vi "USE_THIS_experiment_controller_main_gated.vi"() -> ()   [LabVIEW 2020]
uses:
  <vilib>/Utility/file.llb/Write Delimited Spreadsheet (DBL).vi
  <vilib>/Utility/file.llb/Write To Spreadsheet File (DBL).vi
  <vilib>/Analysis/NI_AALPro.lvlib
  <vilib>/Analysis/2dsp.llb/Integral Method.ctl
  chem-ptch0492/Desktop/IRPD_controler_LV_classic/LeCroy Wave Series/LeCroy Wave Series.lvlib
  <vilib>/Waveform/WDTOps.llb/WDT Get Waveform Subset DBL.vi
panel:
  out "Avg Power / J":dbl format="%#_6f"
  in  "Legacy Mode 2":bool
  in  "Main Tab Control":T1(tab)
  out "Est. total run time / min":dbl
  in  "Legacy Mode":bool
  in  "Scope Trace Tabs":enum32{"Raw Trace", "Avg Traces", "IR Spectrum"}(tab)
  out "Raw Trace":waveform(dbl)(graph)
  out "Avg IR On Chart":waveform(dbl)(graph)
  out "Difference Chart":waveform(dbl)(graph)
  out "Avg IR Off Chart":waveform(dbl)(graph)
  out "Scan Progress":u8(slide) scale=0.0..100.0
  out "IR Spectrum":cluster{dbl[], dbl[]}(graph)
  in  "Laser control":enum32{"Mid IR", "Far IR"}(tab)
  in  "High Position MID / cm-1":dbl
  in  "Step Size MID / cm-1":dbl
  in  "Low Position MID / cm-1":dbl
  in  "Wavenumber MID / cm-1":dbl
  in  "Go to WN MID":bool
  in  "Step Size FAR / cm-1":dbl
  in  "Wavenumber FAR / cm-1":dbl
  in  "High Position FAR / cm-1":dbl
  in  "Low Position FAR / cm-1":dbl
  in  "Go to WN FAR":bool
  in  "Start Scan":bool
  out "Est. time to run / min":dbl
  out "Current Pos / cm-1":dbl
  in  "Number of Sweeps":i32
  in  "Gate Channel (0: Channel 1)":u16(ring) items=["Channel 1", "Channel 2", "Channel 3", "Channel 4", "Memory 1", "Memory 2", "Memory 3", "Memory 4", "Function 1", "Function 2", "Function 3", "Function 4", "Function 5", "Function 6", "Function 7", "Function 8", "Other"]
  in  "Data Channel (0: Channel 1)":u16(ring) items=["Channel 1", "Channel 2", "Channel 3", "Channel 4", "Memory 1", "Memory 2", "Memory 3", "Memory 4", "Function 1", "Function 2", "Function 3", "Function 4", "Function 5", "Function 6", "Function 7", "Function 8", "Other"]
  in  "Laser gate threshold":dbl
  in  "Scope On/Off":bool
  in  "stop":bool
  out "Producer Loop Time / ms":u32
  in  "Auto Setup Scope":bool
  in  "ID Query? (T: Yes)":bool
  in  "Reset? (T: Yes)":bool
  out "Consumer Loop Time / ms":u32
  out "Power / J":dbl
  out "Off queue length":i32
  out "On queue length":i32
  out "Gate Trace":waveform(dbl)(graph)
  out "OPO/OPA motors stationary":bool
  out "OPO/OPA motors reducing errors":bool
  out "OPO/OPA motors scanning red":bool
  out "OPO/OPA motors scanning blue":bool
  # "Ensure that the cursors are gating the peak you are recording the spectrum on if you want a real time spectrum!"
  # "Real Time Controls"
  # "Scanning Controls"
  # "Scan from high to low"
  # "Real Time Controls"
  # "Scanning Controls"
  # "Scan from low to high"
  # "LEAVE THESE ALONE UNLESS YOU KNOW WHAT YOU ARE DOING!"
  # "Gate trace"
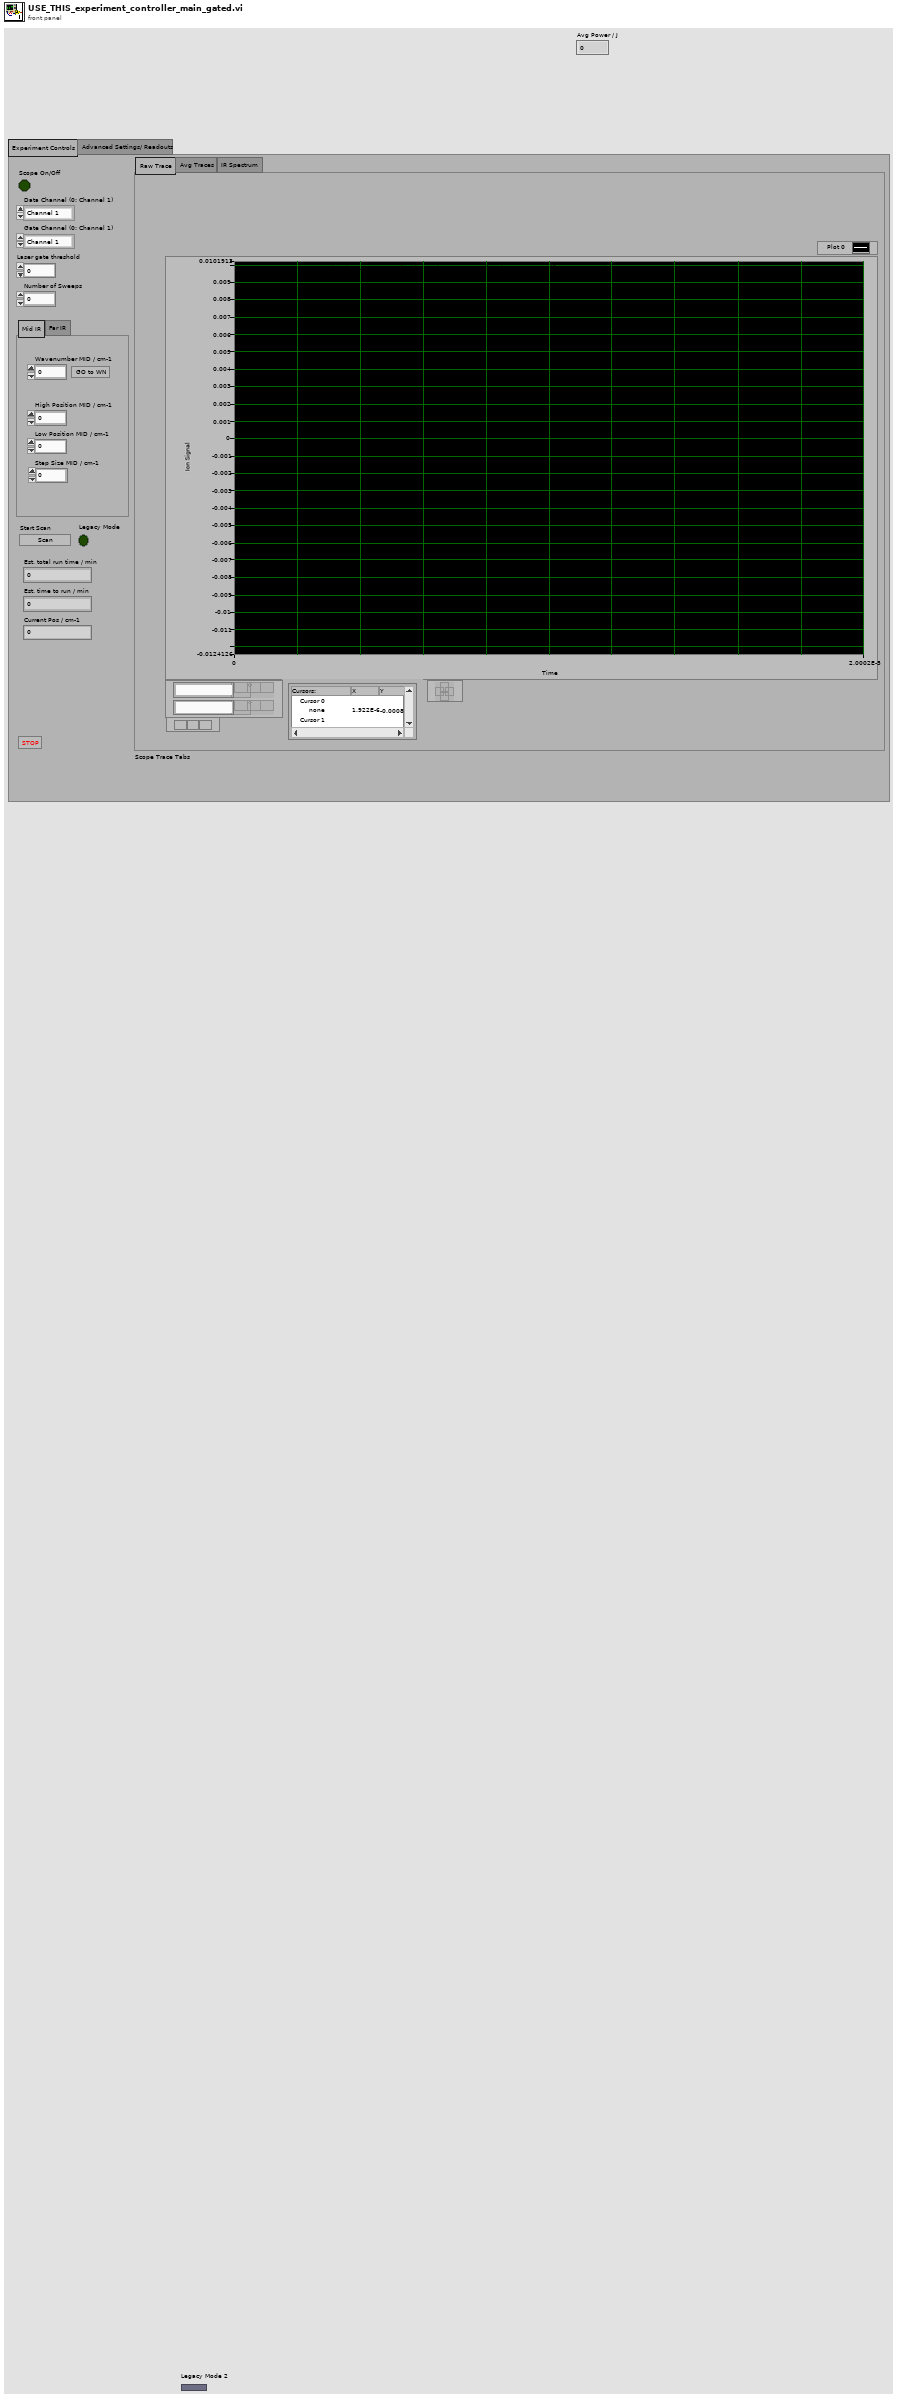
[diagram p1: front panel]
types:
  T1 = enum32{"Experiment Controls", "Advanced Settings/ Readouts"}
  T2 = cluster{"High Position / cm-1":dbl, "Step Size / cm-1":dbl, "Low Position / cm-1":dbl}
  T3 = cluster{"High Position MID / cm-1":dbl, "Step Size MID / cm-1":dbl, "Low Position MID / cm-1":dbl}
  T4 = cluster{"High Position FAR / cm-1":dbl, "Step Size FAR / cm-1":dbl, "Low Position FAR / cm-1 ":dbl}
  T5 = typedef "NI_AALPro.lvlib/Integral Method.ctl" = i32
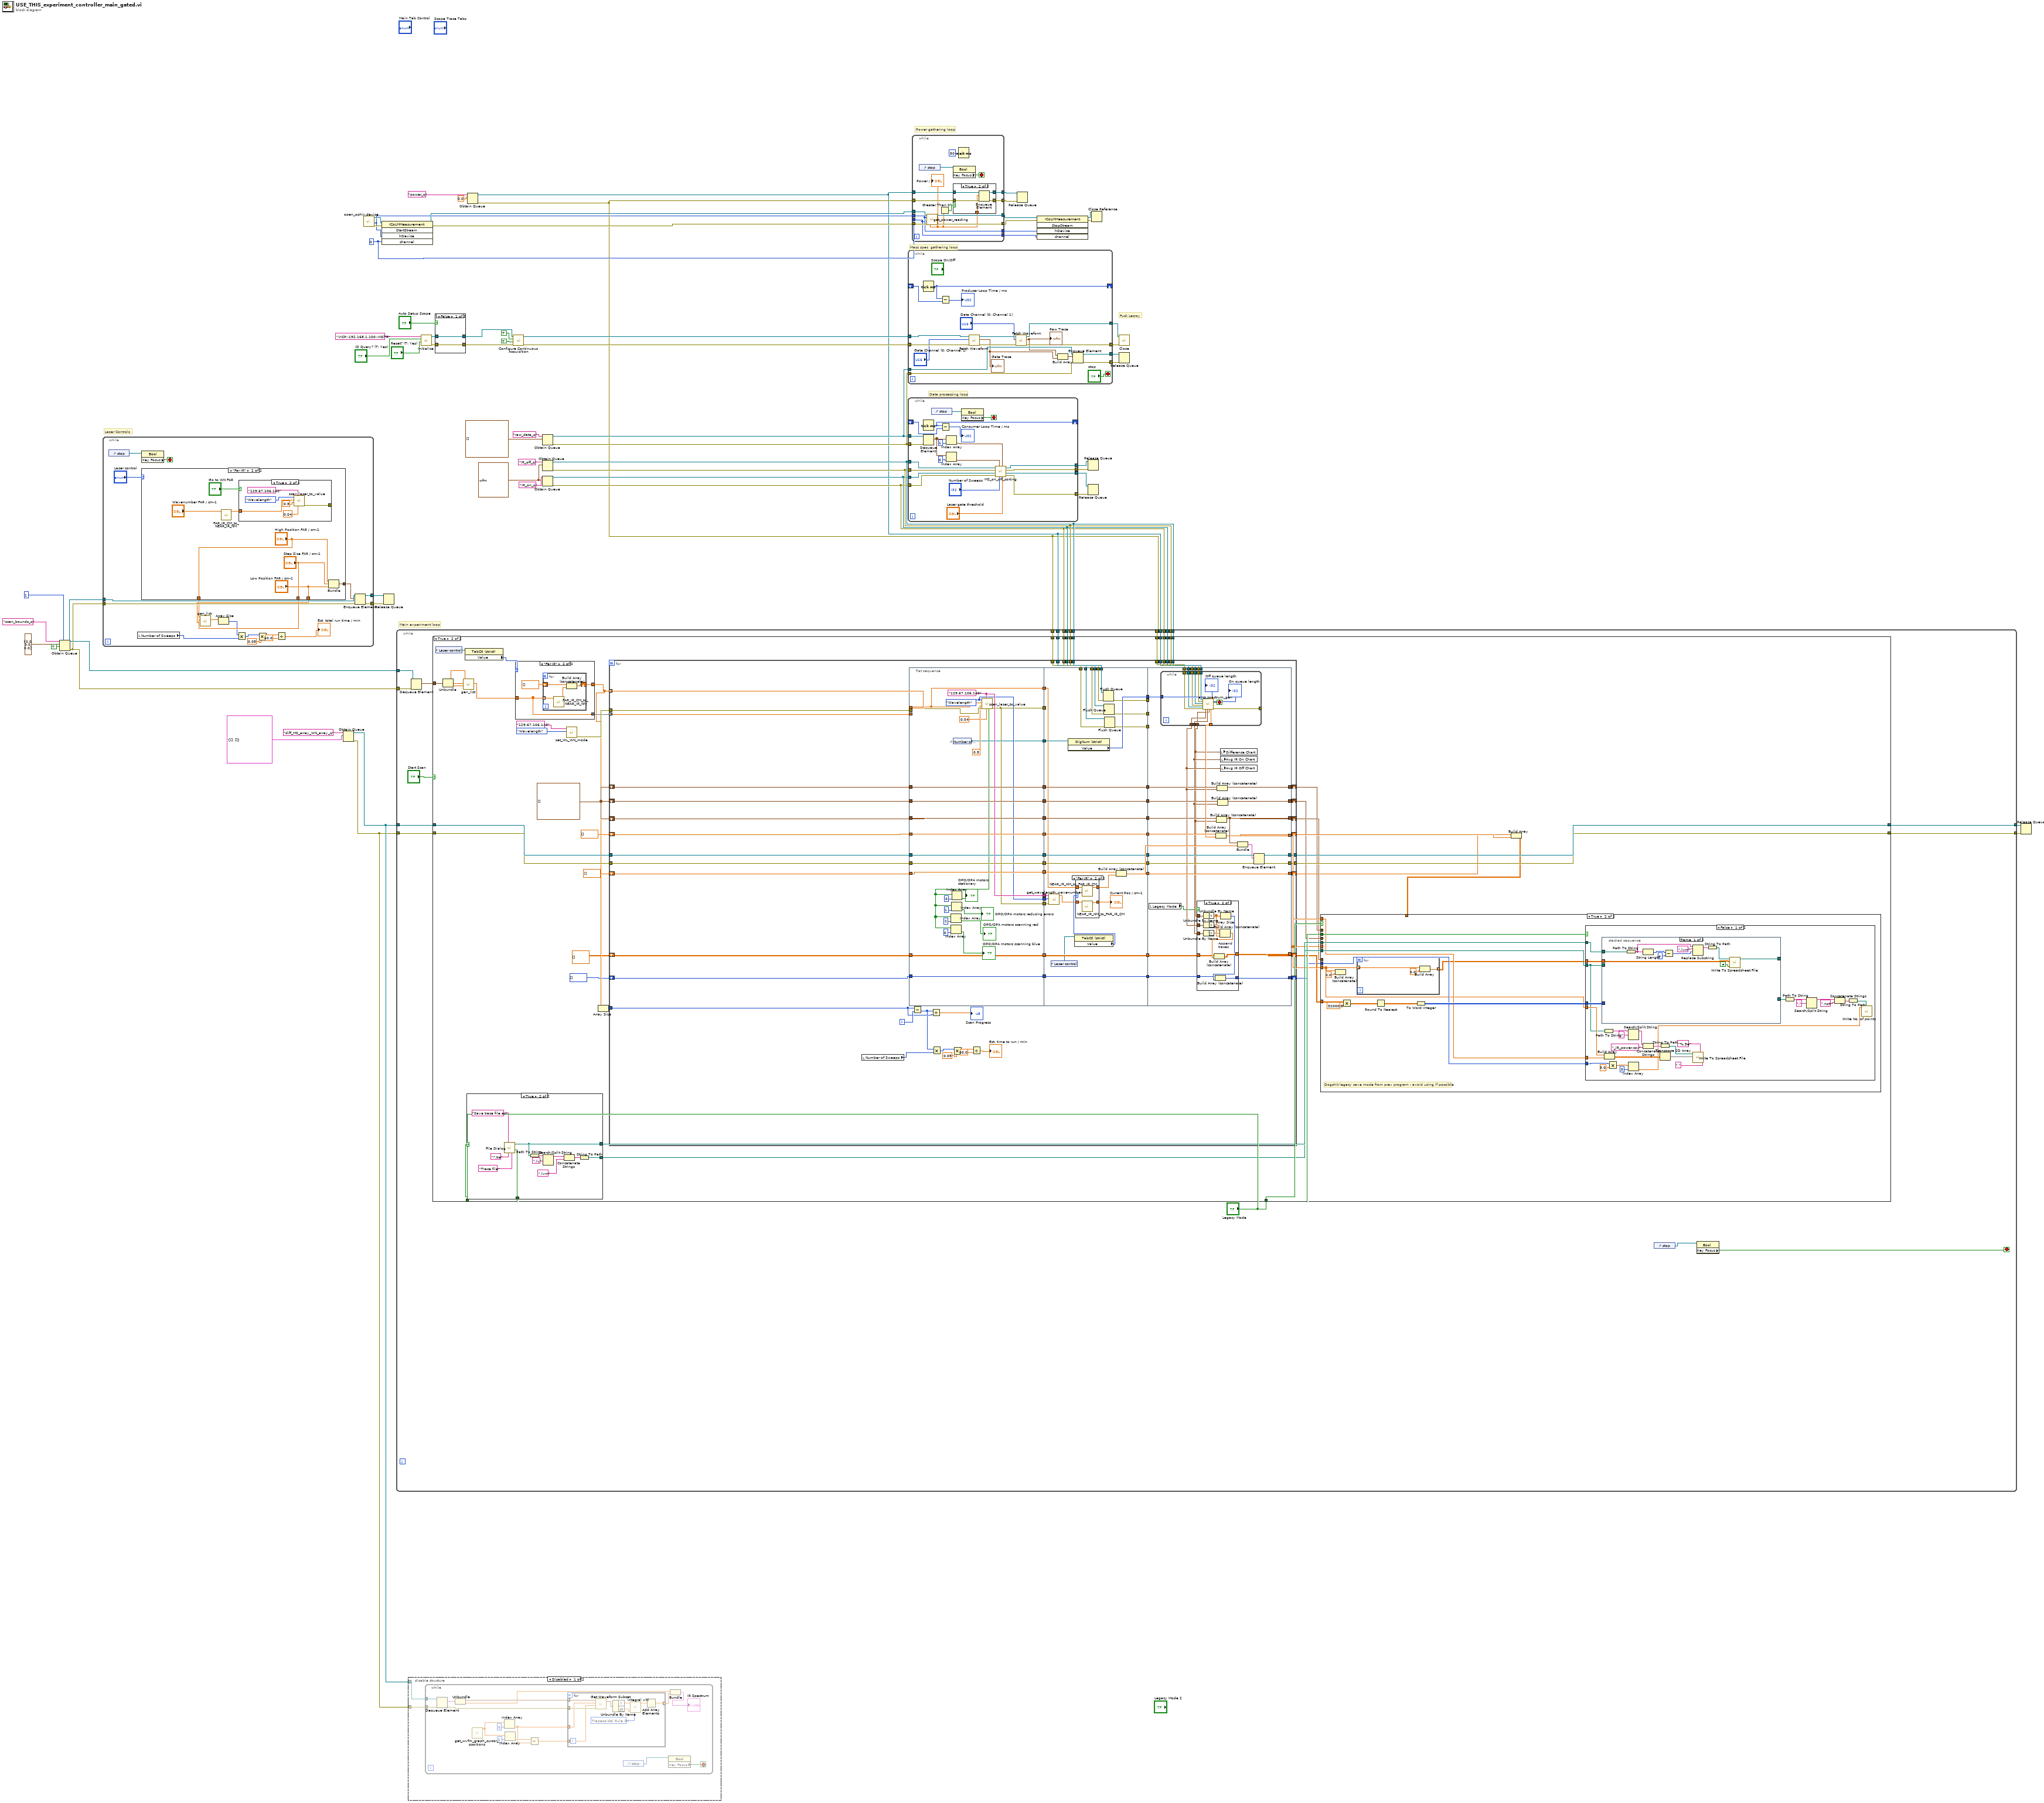
[diagram p0: block diagram]
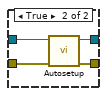
[diagram p3: hidden frame]
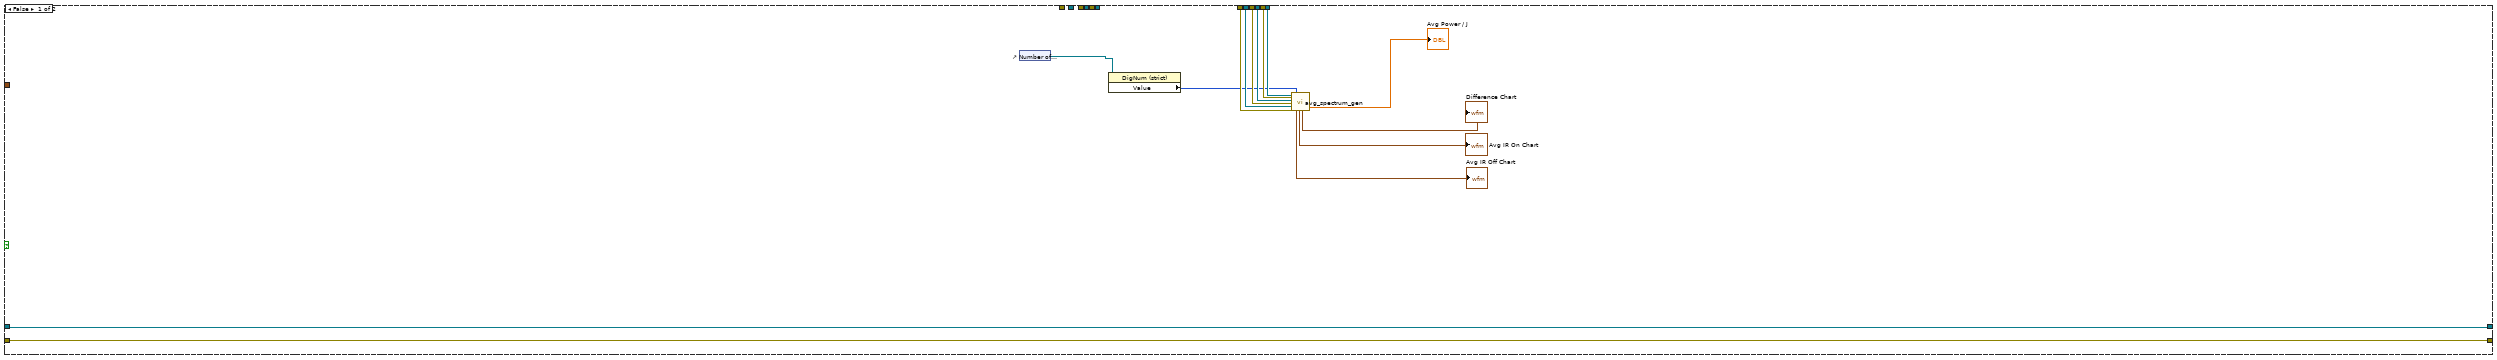
[diagram p5: hidden frame]
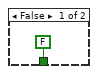
[diagram p6: hidden frame]
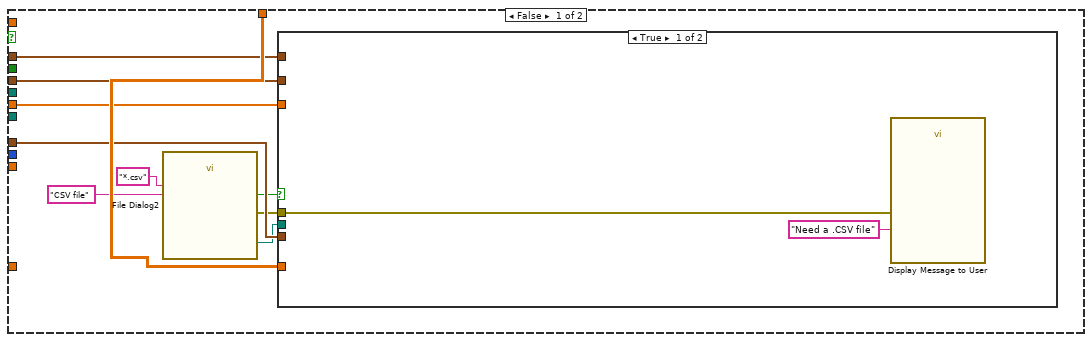
[diagram p7: hidden frame]
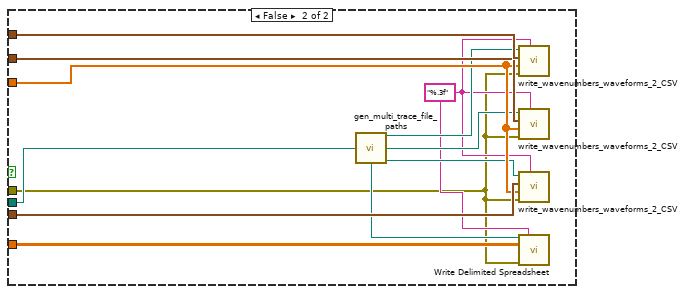
[diagram p8: hidden frame]
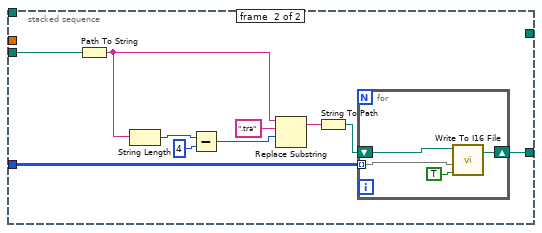
[diagram p9: hidden frame]
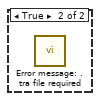
[diagram p10: hidden frame]
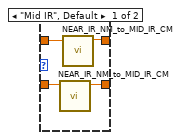
[diagram p11: hidden frame]
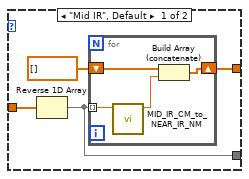
[diagram p13: hidden frame]
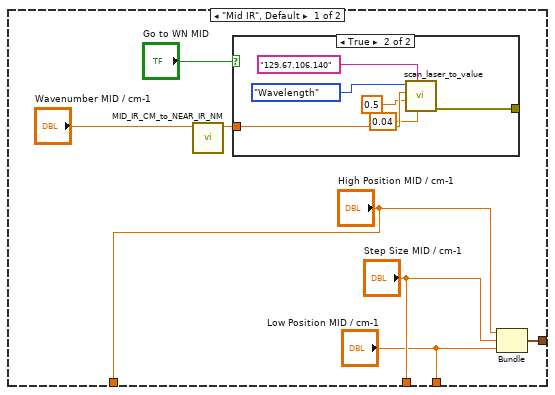
[diagram p14: hidden frame]
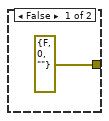
[diagram p15: hidden frame]
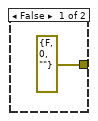
[diagram p16: hidden frame]
diagram:
  w16 = waveform(dbl) {"t0"=timestamp(0 s since 1904-01-01), "dt"=1.0, "Y"=[]} ("element")
  w43 = 0 ("channel")
  # "Fuck Lecroy"
  # "Power gathering loop"
  # "Data processing loop"
  # "Mass spec  gathering loop"
  # "Laser Controls"
  # "Main experiment loop"
  n1 = Obtain Queue(max queue size (-1, unlimited)=1, name (unnamed)="scan_bounds_q", element data type=T2 {"High Position / cm-1"=0.0, "Step Size / cm-1"=0.0, "Low Position / cm-1"=0.0} ("output cluster"), create if not found? (T)=TRUE) -> (queue out=w57:refnum<queue>, error out=w56:errorcluster)  [unwired: 1 in, 1 out]
  n2 = while {
    tunnel: w57 -> [w82]
    tunnel: w56 -> [w81]
    tunnel: [w80] -> w63
    tunnel: [w79] -> w62
    stop <- w76 stop-if-true
    n3 = control-ref of="stop"() -> (w64:refnum<vi>)
    n4 = local read "Number of Sweeps"() -> (w65:i32)
    n5 = property class="Bool"(reference=w64) -> ("Key Focus"=w76:bool)  [unwired: 1 in, 2 out]
    n6 = case shown="\"Far IR\"" "Laser control" {
      tunnel: [w88 w102] -> w77
      tunnel: ["High Position MID / cm-1" "High Position FAR / cm-1"] -> w75
      tunnel: ["Step Size MID / cm-1" "Step Size FAR / cm-1"] -> w74
      tunnel: ["Low Position MID / cm-1" "Low Position FAR / cm-1"] -> w73
      frame "Mid IR", Default {
        n7 = call "MID_IR_CM_to_NEAR_IR_NM.vi"("MID IR / cm-1"="Wavenumber MID / cm-1") -> ("Near IR / nm"=w83:dbl)  [unwired: 10 in]
        n8 = case shown="True" "Go to WN MID" {
          tunnel: w83 -> [_ w94]
          tunnel: [errorcluster {"status"=FALSE, "code"=0, "source"=""} ("error out") w91] -> _
          frame False {
          }
          frame True {
            n9 = call "scan_laser_to_value.vi"("Error range"=0.04, "address"="129.67.106.140", "Scan Speed"=0.5, "Target Value"=w94, "Measure Type"=enum16{"Wavelength", "Wavenumber"}."Wavelength") -> ("error out"=w91:errorcluster)  [unwired: 4 in, 2 out]
          }
        }
        n10 = Bundle("High Position MID / cm-1"="High Position MID / cm-1", "Step Size MID / cm-1"="Step Size MID / cm-1", "Low Position MID / cm-1"="Low Position MID / cm-1") -> (w88:T3)  [unwired: 1 in]
      }
      frame "Far IR" {
        n11 = call "FAR_IR_CM_to_NEAR_IR_NM.vi"("Far IR / cm-1"="Wavenumber FAR / cm-1") -> ("Near IR / nm"=w97:dbl)  [unwired: 10 in]
        n12 = case shown="True" "Go to WN FAR" {
          tunnel: w97 -> [_ w106]
          tunnel: [errorcluster {"status"=FALSE, "code"=0, "source"=""} ("error out") w108] -> _
          frame False {
          }
          frame True {
            n13 = call "scan_laser_to_value.vi"("Error range"=0.04, "address"="129.67.106.140", "Scan Speed"=0.5, "Target Value"=w106, "Measure Type"=enum16{"Wavelength", "Wavenumber"}."Wavelength") -> ("error out"=w108:errorcluster)  [unwired: 4 in, 2 out]
          }
        }
        n14 = Bundle("High Position FAR / cm-1"="High Position FAR / cm-1", "Step Size FAR / cm-1"="Step Size FAR / cm-1", "Low Position FAR / cm-1"="Low Position FAR / cm-1") -> (w102:T4)  [unwired: 1 in]
      }
    }
    n15 = call "gen_list.vi"("Lower Bound"=w73, "Step Size"=w74, "Upper bound"=w75) -> ("Array"=w72:dbl[])  [unwired: 8 in]
    n16 = Array Size(array=w72) -> (size(s)=w71:i32)
    n17 = Multiply(x=w71, y=w65) -> (x*y=w70:i32)
    n18 = Multiply(x=w70, y=0.05) -> (x*y=w68:dbl)
    n19 = Divide(x=w68, y=60.0) -> (x/y=→"Est. total run time / min":dbl)
    n20 = Enqueue Element(queue=w82, element=w77, error in (no error)=w81) -> (queue out=w80:refnum<queue>, error out=w79:errorcluster)  [unwired: 1 in, 1 out]
  }
  n21 = Obtain Queue(name (unnamed)="diff_MS_array_WN_array_q", element data type=cluster{waveform(dbl)[], dbl[]} {[], []} ("output cluster")) -> (queue out=w54:refnum<queue>, error out=w53:errorcluster)  [unwired: 3 in, 1 out]
  n22 = call "open_ophir_device.vi"() -> ("error out"=w48:errorcluster, "hDevice"=w1:i32, "Orphir COM"=w49:refnum<k7>)  [unwired: 7 in, 2 out]
  n23 = invoke class="ICoLMMeasurement" method="StartStream"(reference=w49, error in=w48, "hDevice"=w1, "channel"=w43) -> (reference out=w45:refnum<k7>, error out=w44:errorcluster)  [unwired: 1 in, 3 out]
  n24 = Release Queue(queue=w63, error in (no error)=w62) -> ()  [unwired: 1 in, 3 out]
  n25 = disable-structure shown="Disabled" {
    disable-tunnel: w54 -> [w112 _]
    disable-tunnel: w53 -> [w111 _]
    frame Disabled {
      n26 = while {
        tunnel: w112 -> [w128]
        tunnel: w111 -> [w127]
        stop <- w116 stop-if-true
        n27 = Dequeue Element(queue=w128, error in (no error)=w127) -> (element=w126:cluster{waveform(dbl)[], dbl[]}, error out=w118:errorcluster)  [unwired: 1 in, 2 out]
        n28 = Unbundle(w126) -> (w125:waveform(dbl)[], w117:dbl[])
        n29 = call "get_wvfm_graph_cursor_psoitions.vi"() -> ("X Pos Array"=w124:dbl[])  [unwired: 14 in, 1 out]
        n30 = Index Array(array=w124, index=0) -> (element=w120:dbl)
        n31 = Index Array(array=w124, index=1) -> (element=w121:dbl)
        n32 = Subtract(x=w121, y=w120) -> (x-y=w119:dbl)
        n33 = for {
          tunnel: w125 -> [w138] mode=indexing
          tunnel: w120 -> [w137]
          tunnel: w119 -> [w136]
          tunnel: w118 -> [w135]
          tunnel: [w129] -> w115 mode=indexing
          w131 = T5 0 items=["Trapezoidal Rule", "Simpson's Rule", "Simpson's 3/8 Rule", "Bode Rule"] ("integration method")
          n34 = call-poly <vilib>:"Get Waveform Subset.vi"("error in (no error)"=w135, "duration"=w136, "start samples/time"=w137, "waveform in"=w138) -> ("waveform out"=w134:waveform(dbl))  [unwired: 2 in, 3 out]
          n35 = Unbundle By Name(w134) -> ("Y"=w133:dbl[], "dt"=w132:dbl)
          n36 = call <vilib>:"Integral x(t).vi"("integration method"=w131, "dt"=w132, "X"=w133) -> ("Integral X"=w130:dbl[])  [unwired: 7 in, 1 out]
          n37 = Add Array Elements(numeric array=w130) -> (sum=w129:dbl)
        }
        n38 = control-ref of="stop"() -> (w113:refnum<vi>)
        n39 = property class="Bool"(reference=w113) -> ("Key Focus"=w116:bool)  [unwired: 1 in, 2 out]
        n40 = Bundle(w117, w115) -> (→"IR Spectrum":cluster{dbl[], dbl[]})  [unwired: 1 in]
      }
    }
    frame Enabled {
    }
  }
  n41 = call "Initialize.vi"("Reset? (T: Yes)"="Reset? (T: Yes)", "ID Query? (T: Yes)"="ID Query? (T: Yes)", "VISA resource name"="VICP::192.168.1.100::INSTR") -> ("error out"=w33:errorcluster, "VISA resource name out"=w34:refnum<visa-resource-name>)  [unwired: 7 in]
  n42 = case shown="False" "Auto Setup Scope" {
    tunnel: w34 -> [w140 w144]
    tunnel: w33 -> [w139 w143]
    tunnel: [w140 w142] -> w32
    tunnel: [w139 w141] -> w31
    frame False {
    }
    frame True {
      n43 = call "Autosetup.vi"("error in (no error)"=w143, "VISA resource name"=w144) -> ("error out"=w141:errorcluster, "VISA resource name out"=w142:refnum<visa-resource-name>)  [unwired: 8 in]
    }
  }
  n44 = Obtain Queue(name (unnamed)="power_q", element data type=0.0) -> (queue out=w5:refnum<queue>, error out=w4:errorcluster)  [unwired: 3 in, 1 out]
  n45 = call "Configure Continuous Acquisition.vi"("error in (no error)"=w31, "Auto Trigger Enabled (T: Normal)"=TRUE, "Continuous Acquisition Mode (T: On)"=TRUE, "VISA resource name"=w32) -> ("error out"=w27:errorcluster, "VISA resource name out"=w28:refnum<visa-resource-name>)  [unwired: 6 in]
  n46 = Obtain Queue(name (unnamed)="raw_data_q", element data type=waveform(dbl)[] [] ("appended array")) -> (queue out=w11:refnum<queue>, error out=w10:errorcluster)  [unwired: 3 in, 1 out]
  n47 = Obtain Queue(name (unnamed)="IR_off_q", element data type=w16) -> (queue out=w9:refnum<queue>, error out=w8:errorcluster)  [unwired: 3 in, 1 out]
  n48 = Obtain Queue(name (unnamed)="IR_on_q", element data type=w16) -> (queue out=w7:refnum<queue>, error out=w6:errorcluster)  [unwired: 3 in, 1 out]
  n49 = while {
    tunnel: w57 -> [w167]
    tunnel: w56 -> [w166]
    tunnel: w54 -> [w162]
    tunnel: w53 -> [w161]
    tunnel: [w160] -> w51
    tunnel: [w159] -> w50
    tunnel: w9 -> [w157]
    tunnel: w8 -> [w156]
    tunnel: w7 -> [w155]
    tunnel: w6 -> [w154]
    tunnel: w5 -> [w153]
    tunnel: w4 -> [w152]
    tunnel: w9 -> [w151]
    tunnel: w8 -> [w150]
    tunnel: w7 -> [w149]
    tunnel: w6 -> [w148]
    tunnel: w5 -> [w147]
    tunnel: w4 -> [w146]
    stop <- w165 stop-if-true
    n50 = Dequeue Element(queue=w167, error in (no error)=w166) -> (element=w164:T2)  [unwired: 1 in, 3 out]
    n51 = case shown="True" "Start Scan" {
      tunnel: w164 -> [_ w228]
      tunnel: w162 -> [w181 w217]
      tunnel: w161 -> [w180 w216]
      tunnel: [w181 w215] -> w160
      tunnel: [w180 w214] -> w159
      tunnel: "Legacy Mode" -> [_ w210]
      tunnel: "Legacy Mode" -> [_ w205]
      tunnel: w157 -> [w176 w193]
      tunnel: w156 -> [w175 w192]
      tunnel: w155 -> [w174 w191]
      tunnel: w154 -> [w173 w190]
      tunnel: w153 -> [w172 w189]
      tunnel: w152 -> [w171 w188]
      tunnel: w151 -> [_ w187]
      tunnel: w150 -> [_ w186]
      tunnel: w149 -> [_ w185]
      tunnel: w148 -> [_ w184]
      tunnel: w147 -> [_ w183]
      tunnel: w146 -> [_ w182]
      frame False {
        n52 = control-ref of="Number of Sweeps"() -> (w170:refnum<vi>)
        n53 = property class="DigNum (strict)"(reference=w170) -> ("Value"=w169:i32)  [unwired: 1 in, 2 out]
        n54 = call "avg_spectrum_gen.vi"("IR_off_q_in"=w176, "IR_off_q_error_in"=w175, "IR_on_q_in"=w174, "IR_on_q_error_in"=w173, "power_q_in"=w172, "power_q_error_in"=w171, "Number of sweeps"=w169) -> ("Avg Off Trace"=→"Avg IR Off Chart":waveform(dbl), "Avg On Trace"=→"Avg IR On Chart":waveform(dbl), "Difference Trace"=→"Difference Chart":waveform(dbl), "Avg Power / J"=→"Avg Power / J":dbl)  [unwired: 9 out]
      }
      frame True {
        w218 = waveform(dbl)[] [] ("waveform array")
        n55 = control-ref of="Laser control"() -> (w224:refnum<vi>)
        n56 = Unbundle(w228) -> ("High Position / cm-1"=w227:dbl, "Step Size / cm-1"=w226:dbl, "Low Position / cm-1"=w225:dbl)
        n57 = call "gen_list.vi"("Lower Bound"=w225, "Step Size"=w226, "Upper bound"=w227) -> ("Array"=w222:dbl[])  [unwired: 8 in]
        n58 = property class="TabCtl (strict)"(reference=w224) -> ("Value"=w223:enum32{"Mid IR", "Far IR"})  [unwired: 1 in, 2 out]
        n59 = case shown="True" w205 {
          tunnel: [_ w236] -> w209
          tunnel: [_ w232] -> w208
          tunnel: [FALSE ("cancelled") w231] -> w206
          frame False {
          }
          frame True {
            n60 = call "File Dialog"("prompt"="Save trace file as", "pattern (all files)"="*.tra", "pattern label"="Trace file") -> ("selected path"=w236:path, "cancelled"=w231:bool)  [unwired: 9 in, 2 out]
            n61 = Path To String(path=w236) -> (string=w237:string)
            n62 = Search/Split String(string=w237, search string/char (-)=".lv") -> (substring before match=w235:string)  [unwired: 1 in, 2 out]
            n63 = Concatenate Strings(w235, ".lvm" ("string")) -> (w233:string)
            n64 = String To Path(string=w233) -> (path=w232:path)
          }
        }
        n65 = case shown="\"Far IR\"" w223 {
          tunnel: w222 -> [w531 w536]
          tunnel: [w529 w537] -> w199
          tunnel: [w528 w536] -> w211
          frame "Mid IR", Default {
            n66 = Reverse 1D Array(array=w531) -> (reversed array=w528:dbl[])
            n67 = for {
              tunnel: w528 -> [w533] mode=indexing
              shift-right: [w535] -> w529
              shift-left: dbl[] [] -> [w534]
              n68 = call "MID_IR_CM_to_NEAR_IR_NM.vi"("MID IR / cm-1"=w533) -> ("Near IR / nm"=w532:dbl)  [unwired: 10 in]
              n69 = Build Array (concatenate)(w534, w532) -> (w535:dbl[])
            }
          }
          frame "Far IR" {
            n70 = for {
              tunnel: w536 -> [w539] mode=indexing
              shift-right: [w542] -> w537
              shift-left: dbl[] [] -> [w541]
              n71 = call "FAR_IR_CM_to_NEAR_IR_NM.vi"("Far IR / cm-1"=w539) -> ("Near IR / nm"=w540:dbl)  [unwired: 10 in]
              n72 = Build Array (concatenate)(w541, w540) -> (w542:dbl[])
            }
          }
        }
        n73 = call "set_WL_WN_mode.vi"("Measure Type"=enum16{"Wavelength", "Wavenumber"}."Wavelength", "address"="129.67.106.140") -> ("error out"=w219:errorcluster)  [unwired: 9 in]
        n74 = Array Size(array=w199) -> (size(s)=w198:i32)
        n75 = for {
          tunnel: w199 -> [w404] mode=indexing
          tunnel: w219 -> [w403]
          shift-right: [w393] -> w204
          shift-left: w218 -> [w402]
          shift-right: [w392] -> w203
          shift-left: w218 -> [w397]
          shift-right: [w391] -> w202
          shift-left: w218 -> [w396]
          tunnel: w217 -> [w388]
          tunnel: w216 -> [w386]
          tunnel: [w383] -> w215
          tunnel: [w382] -> w214
          shift-right: [w353] -> w201
          shift-left: dbl[] [] ("appended array") -> [w366]
          shift-right: [w377] -> w207
          shift-left: dbl[] [] ("appended array") -> [w378]
          tunnel: w211 -> [w376] mode=indexing
          tunnel: w198 -> [w374]
          shift-right: [w361] -> w196
          shift-left: dbl[][] [] -> [w362]
          shift-right: [w360] -> w194
          shift-left: i32[] [] -> [w358]
          tunnel: w193 -> [w352]
          tunnel: w192 -> [w351]
          tunnel: w191 -> [w350]
          tunnel: w190 -> [w349]
          tunnel: w189 -> [w348]
          tunnel: w188 -> [w347]
          tunnel: w187 -> [w346]
          tunnel: w186 -> [w345]
          tunnel: w185 -> [w344]
          tunnel: w184 -> [w343]
          tunnel: w183 -> [w342]
          tunnel: w182 -> [w341]
          i -> [w375]
          n76 = local read "Number of Sweeps"() -> (w339:i32)
          n77 = flat-sequence {
            tunnel: w404 -> [w415]
            tunnel: w403 -> [w430]
            tunnel: w402 -> [w429]
            tunnel: [w429] -> w400
            tunnel: [w428] -> w398
            tunnel: w397 -> [w428]
            tunnel: w396 -> [w427]
            tunnel: [w427] -> w394
            tunnel: [w426] -> w389
            tunnel: w388 -> [w426]
            tunnel: w386 -> [w425]
            tunnel: [w425] -> w384
            tunnel: w378 -> [w424]
            tunnel: [w424] -> w380
            tunnel: w376 -> [_]
            tunnel: w366 -> [w421]
            tunnel: [w421] -> w365
            tunnel: w362 -> [w420]
            tunnel: [w420] -> w363
            tunnel: w358 -> [w419]
            tunnel: [w419] -> w357
            tunnel: [w418] -> w356
            tunnel: [w417] -> w355
            tunnel: [w414] -> w354
            tunnel: [w416] -> w340
            tunnel: [w415] -> w338
            tunnel: [w414] -> w337
            tunnel: [w460] -> w401
            tunnel: w400 -> [w460]
            tunnel: [w459] -> w399
            tunnel: w398 -> [w459]
            tunnel: [w458] -> w395
            tunnel: w394 -> [w458]
            tunnel: [w457] -> w390
            tunnel: w389 -> [w456]
            tunnel: [w456] -> w387
            tunnel: [w455] -> w385
            tunnel: w384 -> [w455]
            tunnel: [w453] -> w381
            tunnel: w380 -> [w454]
            tunnel: [w454] -> w379
            tunnel: w365 -> [w452]
            tunnel: [w451] -> w364
            tunnel: w363 -> [w451]
            tunnel: [w450] -> w359
            tunnel: w357 -> [w450]
            tunnel: w356 -> [w449]
            tunnel: w355 -> [w448]
            tunnel: w354 -> [w447]
            tunnel: w346 -> [w442]
            tunnel: w345 -> [w441]
            tunnel: w344 -> [w440]
            tunnel: w343 -> [w439]
            tunnel: w342 -> [w438]
            tunnel: w341 -> [w437]
            tunnel: w340 -> [w436]
            tunnel: w338 -> [w432]
            tunnel: w337 -> [_]
            tunnel: [w435] -> w336
            tunnel: [w434] -> w335
            tunnel: [w433] -> w334
            tunnel: [w497] -> w393
            tunnel: w401 -> [w498]
            tunnel: [w495] -> w392
            tunnel: w399 -> [w496]
            tunnel: [w488] -> w391
            tunnel: w395 -> [w494]
            tunnel: w390 -> [w493]
            tunnel: w387 -> [w492]
            tunnel: w385 -> [w491]
            tunnel: [w490] -> w383
            tunnel: [w489] -> w382
            tunnel: w381 -> [w487]
            tunnel: [w487] -> w353
            tunnel: w379 -> [w486]
            tunnel: [w485] -> w377
            tunnel: w364 -> [w479]
            tunnel: [w478] -> w361
            tunnel: [w477] -> w360
            tunnel: w359 -> [w476]
            tunnel: w352 -> [w474]
            tunnel: w351 -> [w473]
            tunnel: w350 -> [w472]
            tunnel: w349 -> [w471]
            tunnel: w348 -> [w470]
            tunnel: w347 -> [w469]
            tunnel: w336 -> [_]
            tunnel: w335 -> [_]
            tunnel: w334 -> [_]
            frame #0 {
              w417 = enum16{"Wavelength", "Wavenumber"}."Wavelength" ("Measure Type")
              w418 = "129.67.106.140" ("address")
              n78 = control-ref of="Number of Sweeps"() -> (w416:refnum<vi>)
              n79 = call "scan_laser_to_value.vi"("Error range"=0.04, "address"=w418, "error in"=w430, "Scan Speed"=0.5, "Target Value"=w415, "Measure Type"=w417) -> ("error out"=w414:errorcluster, "Motor status array"=w413:bool[])  [unwired: 3 in, 1 out]
              n80 = Index Array(array=w413, index=0) -> (element=→"OPO/OPA motors scanning blue":bool)
              n81 = Index Array(array=w413, index=2) -> (element=→"OPO/OPA motors scanning red":bool)
              n82 = Index Array(array=w413, index=1) -> (element=→"OPO/OPA motors reducing errors":bool)
              n83 = Index Array(array=w413, index=0) -> (element=→"OPO/OPA motors stationary":bool)
            }
            frame #1 {
              n84 = call "get_wavelength_wavenumber.vi"("error in"=w447, "Measure Type"=w448, "address"=w449) -> ("Wavelength/Wavenuumber"=w444:dbl)  [unwired: 7 in, 1 out]
              n85 = control-ref of="Laser control"() -> (w445:refnum<vi>)
              n86 = property class="DigNum (strict)"(reference=w436) -> ("Value"=w457:i32)  [unwired: 1 in, 2 out]
              n87 = property class="TabCtl (strict)"(reference=w445) -> ("Value"=w446:enum32{"Mid IR", "Far IR"})  [unwired: 1 in, 2 out]
              n88 = case shown="\"Far IR\"" w446 {
                tunnel: w444 -> [w464 w468]
                tunnel: [w463 w467] -> w443
                tunnel: w432 -> [w462 w466]
                tunnel: [w461 w465] -> w431
                frame "Mid IR", Default {
                  n89 = call "NEAR_IR_NM_to_MID_IR_CM.vi"("Near IR / nm"=w464) -> ("MID IR / cm-1"=w463:dbl)  [unwired: 10 in]
                  n90 = call "NEAR_IR_NM_to_MID_IR_CM.vi"("Near IR / nm"=w462) -> ("MID IR / cm-1"=w461:dbl)  [unwired: 10 in]
                }
                frame "Far IR" {
                  n91 = call "NEAR_IR_NM_to_FAR_IR_CM.vi"("Near IR / nm"=w466) -> ("Far IR / cm-1"=w465:dbl)  [unwired: 10 in]
                  n92 = call "NEAR_IR_NM_to_FAR_IR_CM.vi"("Near IR / nm"=w468) -> ("Far IR / cm-1"=w467:dbl)  [unwired: 10 in]
                }
              }
              "Current Pos / cm-1" <- w443
              n93 = Flush Queue(queue=w442, error in (no error)=w441) -> (error out=w435:errorcluster)  [unwired: 2 out]
              n94 = Flush Queue(queue=w440, error in (no error)=w439) -> (error out=w434:errorcluster)  [unwired: 2 out]
              n95 = Flush Queue(queue=w438, error in (no error)=w437) -> (error out=w433:errorcluster)  [unwired: 2 out]
              n96 = Build Array (concatenate)(w452, w431) -> (w453:dbl[])
            }
            frame #2 {
              n97 = local read "Legacy Mode"() -> (w480:bool)
              n98 = while {
                tunnel: [w527] -> w483
                tunnel: [w526] -> w482
                tunnel: [w525] -> w481
                tunnel: w493 -> [w523]
                tunnel: [w522] -> w484
                tunnel: w474 -> [w521]
                tunnel: w473 -> [w520]
                tunnel: w472 -> [w519]
                tunnel: w471 -> [w518]
                tunnel: w470 -> [w517]
                tunnel: w469 -> [w516]
                tunnel: [w515] -> _
                stop <- w524 stop-if-true
                n99 = call "avg_spectrum_gen.vi"("IR_off_q_in"=w521, "IR_off_q_error_in"=w520, "IR_on_q_in"=w519, "IR_on_q_error_in"=w518, "power_q_in"=w517, "power_q_error_in"=w516, "Number of sweeps"=w523) -> ("Avg Off Trace"=w527:waveform(dbl), "Off queue length"=→"Off queue length":i32, "Avg On Trace"=w526:waveform(dbl), "On queue length"=→"On queue length":i32, "Difference Trace"=w525:waveform(dbl), "Finished Gathering"=w524:bool, "Avg Power / J"=w522:dbl, "power_q_error_out"=w515:errorcluster)  [unwired: 5 out]
              }
              n100 = case shown="True" w480 {
                tunnel: w483 -> [_ w510]
                tunnel: w482 -> [_ w509]
                tunnel: w481 -> [_ w508]
                tunnel: [w500 w505] -> w478
                tunnel: w479 -> [w500 w504]
                tunnel: [w499 w502] -> w477
                tunnel: w476 -> [w499 w501]
                frame False {
                }
                frame True {
                  n101 = Unbundle By Name(w508) -> ("Y"=w507:dbl[])
                  n102 = Unbundle By Name(w510) -> ("Y"=w512:dbl[])
                  n103 = Unbundle By Name(w509) -> ("Y"=w511:dbl[])
                  n104 = Build Array (concatenate) "Append \ntraces"(w512, w511, w507) -> (w506:dbl[])
                  n105 = Build Array (concatenate)(w504, w506) -> (w505:dbl[][])
                  n106 = Array Size(array=w507) -> (size(s)=w503:i32)
                  n107 = Build Array (concatenate)(w501, w503) -> (w502:i32[])
                }
              }
              n108 = Build Array (concatenate)(w486, w484) -> (w485:dbl[])
              n109 = Build Array (concatenate)(w494, w481) -> (w488:waveform(dbl)[])
              n110 = Build Array (concatenate)(w498, w483) -> (w497:waveform(dbl)[])
              n111 = Build Array (concatenate)(w496, w482) -> (w495:waveform(dbl)[])
              n112 = local write "Difference Chart"(w481) -> ()
              n113 = local write "Avg IR On Chart"(w482) -> ()
              n114 = local write "Avg IR Off Chart"(w483) -> ()
              n115 = Bundle(w488, w487) -> (w475:cluster{waveform(dbl)[], dbl[]})  [unwired: 1 in]
              n116 = Enqueue Element(queue=w492, element=w475, error in (no error)=w491) -> (queue out=w490:refnum<queue>, error out=w489:errorcluster)  [unwired: 1 in, 1 out]
            }
          }
          n117 = Subtract(x=w374, y=w375) -> (x-y=w368:i32)
          n118 = Divide(x=w368, y=w374) -> (x/y=→"Scan Progress":dbl)
          n119 = Multiply(x=w368, y=w339) -> (x*y=w372:i32)
          n120 = Multiply(x=w372, y=0.05) -> (x*y=w370:dbl)
          n121 = Divide(x=w370, y=60.0) -> (x/y=→"Est. time to run / min":dbl)
        }
        n122 = Build Array(w201, w207) -> (w200:dbl[][])
        n123 = case shown="True" w210 {
          tunnel: w201 -> [_ w267]
          tunnel: w209 -> [_ w269]
          tunnel: w208 -> [_ w272]
          tunnel: w206 -> [_ w271]
          tunnel: w194 -> [_ w270]
          tunnel: w207 -> [_ w268]
          tunnel: w200 -> [w250 _]
          tunnel: w204 -> [w249 _]
          tunnel: w203 -> [w248 _]
          tunnel: w202 -> [w247 _]
          tunnel: w201 -> [w246 _]
          tunnel: w196 -> [_ w265]
          frame False {
            n124 = call "File Dialog2"("pattern (all files)"="*.csv", "pattern label"="CSV file") -> ("selected path"=w241:path, "cancelled"=w243:bool, "error out"=w242:errorcluster)  [unwired: 10 in, 1 out]
            n125 = case shown="True" w243 {
              tunnel: w241 -> [_ w260]
              tunnel: w250 -> [_ w256]
              tunnel: w249 -> [_ w264]
              tunnel: w248 -> [_ w263]
              tunnel: w247 -> [_ w262]
              tunnel: w246 -> [_ w261]
              tunnel: w242 -> [w251 w253]
              frame True {
                n126 = call "Display Message to User"("error in (no error)"=w251, "Message"="Need a .CSV file") -> ()  [unwired: 8 in, 2 out]
              }
              frame False {
                w254 = "%.3f" ("format (%.3f)")
                n127 = call "gen_multi_trace_file_paths.vi"("Generic trace file path"=w260) -> ("avg_IR_off_path"=w259:path, "avg_IR_on_path"=w258:path, "avg_IR_power_path"=w255:path, "avg_diff_path"=w257:path)  [unwired: 11 in]
                n128 = call "write_wavenumbers_waveforms_2_CSV.vi"("format (%.3f)"=w254, "error in (no error)"=w253, "Wavenumber Array"=w261, "Waveform Array"=w264, "file path (dialog if empty)"=w259) -> ()  [unwired: 6 in, 1 out]
                n129 = call "write_wavenumbers_waveforms_2_CSV.vi"("format (%.3f)"=w254, "error in (no error)"=w253, "Wavenumber Array"=w261, "Waveform Array"=w263, "file path (dialog if empty)"=w258) -> ()  [unwired: 6 in, 1 out]
                n130 = call "write_wavenumbers_waveforms_2_CSV.vi"("format (%.3f)"=w254, "error in (no error)"=w253, "Wavenumber Array"=w261, "Waveform Array"=w262, "file path (dialog if empty)"=w257) -> ()  [unwired: 6 in, 1 out]
                n131 = call-poly <vilib>:"Write Delimited Spreadsheet.vi"("file path (dialog if empty)"=w255, "format (%.3f)"=w254, "2D data"=w256, "error in (no error)"=w253) -> ()  [unwired: 10 in, 2 out]
              }
            }
          }
          frame True {
            # "Dogshit legacy save mode from prev program - avoid using if possible"
            n132 = Build Array (concatenate)(w267, 0.0) -> ()  [unwired: 1 out]
            n133 = Multiply(x=w265, y=32000.0) -> (x*y=w276:dbl[][])
            n134 = for {
              tunnel: w267 -> [w280] mode=indexing
              tunnel: [w278] -> w266 mode=indexing
              n135 = Build Array(w280, 0.0) -> (w278:dbl[])
            }
            n136 = Round To Nearest(number=w276) -> (nearest integer value=w277:dbl[][])
            n137 = To Word Integer(number=w277) -> (16bit integer=w274:i16[][])
            n138 = case shown="False" w271 {
              tunnel: w274 -> [w308 _]
              tunnel: w269 -> [w286 _]
              tunnel: w272 -> [w307 _]
              tunnel: w270 -> [w298 _]
              tunnel: w267 -> [w291 _]
              tunnel: w268 -> [w290 _]
              tunnel: w266 -> [w281 _]
              frame False {
                n139 = stacked-sequence {
                  tunnel: [_ w329] -> w306
                  tunnel: w286 -> [_ w322]
                  tunnel: w308 -> [_ w320]
                  tunnel: [w314 _] -> _
                  tunnel: w307 -> [w313 _]
                  tunnel: w281 -> [w309 _]
                  frame #0 {
                    n140 = Path To String(path=w313) -> (string=w312:string)
                    n141 = String Length(string=w312) -> (length=w319:i32)
                    n142 = Subtract(x=w319, y=4) -> (x-y=w317:i32)
                    n143 = Replace Substring(3:w317, 4:".lvm" ("substring (\"\")"), 5:w312) -> (1:w316:string)  [unwired: 1 in, 1 out]
                    n144 = String To Path(string=w316) -> (path=w315:path)
                    n145 = call-poly <vilib>:"Write To Spreadsheet File.vi"("append to file? (new file:F)"=FALSE, "2D data"=w309, "file path (dialog if empty)"=w315) -> ("new file path (Not A Path if cancelled)"=w314:path)  [unwired: 5 in]
                  }
                  frame #1 {
                    n146 = Path To String(path=w322) -> (string=w325:string)
                    n147 = String Length(string=w325) -> (length=w328:i32)
                    n148 = Subtract(x=w328, y=4) -> (x-y=w326:i32)
                    n149 = Replace Substring(3:w326, 4:".tra" ("substring (\"\")"), 5:w325) -> (1:w324:string)  [unwired: 1 in, 1 out]
                    n150 = String To Path(string=w324) -> (path=w323:path)
                    n151 = for {
                      shift-right: [w332] -> w329
                      shift-left: w323 -> [w331]
                      tunnel: w320 -> [w330] mode=indexing
                      n152 = call <vilib>:"Write To I16 File.vi"("append to file? (new file:F)"=TRUE, "1D array"=w330, "file path (dialog if empty)"=w331) -> ("new file path (Not A Path if cancelled)"=w332:path)  [unwired: 4 in]
                    }
                  }
                }
                n153 = Path To String(path=w286) -> (string=w292:string)
                n154 = Build Array(w291, w290) -> (w296:dbl[][])
                n155 = Multiply(x=w298, y=3.0) -> (x*y=w282:dbl[])
                n156 = Index Array(array=w282, index=0) -> (element=w283:dbl)
                n157 = Search/Split String(string=w292, search string/char (-)=".") -> (substring before match=w293:string)  [unwired: 1 in, 2 out]
                n158 = Concatenate Strings(w293, "_IR_power.csv" ("string")) -> (w294:string)
                n159 = String To Path(string=w294) -> (path=w295:path)
                n160 = Transpose 2D Array(2D array=w296) -> (transposed array=w297:dbl[][])
                n161 = call-poly <vilib>:"Write To Spreadsheet File.vi"("delimiter (\\t)"="," ("delimiter (\\t)"), "format (%.3f)"="%.5e", "2D data"=w297, "file path (dialog if empty)"=w295) -> ()  [unwired: 4 in, 1 out]
                n162 = Path To String(path=w306) -> (string=w305:string)
                n163 = Search/Split String(string=w305, search string/char (-)=".") -> (substring before match=w303:string)  [unwired: 1 in, 2 out]
                n164 = Concatenate Strings(w303, ".npt" ("string")) -> (w301:string)
                n165 = String To Path(string=w301) -> (path=w300:path)
                n166 = call "Write No. of points"("Signals"=w283, "File Name"=w300) -> ()  [unwired: 15 in, 3 out]
              }
              frame True {
                n167 = call "Error message: .tra file required"() -> ()  [unwired: 10 in, 2 out]
              }
            }
          }
        }
      }
    }
    n168 = control-ref of="stop"() -> (w145:refnum<vi>)
    n169 = property class="Bool"(reference=w145) -> ("Key Focus"=w165:bool)  [unwired: 1 in, 2 out]
  }
  n170 = while {
    tunnel: w28 -> [w552]
    tunnel: w27 -> [w551]
    tunnel: [w561] -> w25
    tunnel: [w560] -> w24
    tunnel: w11 -> [w550]
    tunnel: [w548] -> w13
    tunnel: w10 -> [w549]
    tunnel: [w547] -> w12
    shift-right: [w558] -> _
    shift-left: _ -> [w559]
    stop <- "stop" stop-if-true
    n171 = Tick Count (ms)() -> (millisecond timer value=w558:u32)
    n172 = Subtract(x=w558, y=w559) -> (x-y=→"Producer Loop Time / ms":u32)
    n173 = call "Fetch Waveform.vi"("error in (no error)"=w551, "Source (0: Channel 1)"="Gate Channel (0: Channel 1)", "VISA resource name"=w552) -> ("error out"=w553:errorcluster, "Waveform Graph"=w545:waveform(dbl), "VISA resource name out"=w554:refnum<visa-resource-name>)  [unwired: 6 in]
    "Gate Trace" <- w545
    n174 = call "Fetch Waveform.vi"("error in (no error)"=w553, "Source (0: Channel 1)"="Data Channel (0: Channel 1)", "VISA resource name"=w554) -> ("error out"=w560:errorcluster, "Waveform Graph"=w546:waveform(dbl), "VISA resource name out"=w561:refnum<visa-resource-name>)  [unwired: 6 in]
    "Raw Trace" <- w546
    n175 = Build Array(w546, w545) -> (w544:waveform(dbl)[])
    n176 = Enqueue Element(queue=w550, element=w544, error in (no error)=w549) -> (queue out=w548:refnum<queue>, error out=w547:errorcluster)  [unwired: 1 in, 1 out]
  }
  n177 = while {
    tunnel: w9 -> [w579]
    tunnel: w8 -> [w577]
    tunnel: w7 -> [w578]
    tunnel: w6 -> [w576]
    shift-right: [w580] -> _
    shift-left: _ -> [w581]
    tunnel: [w575] -> w15
    tunnel: [w574] -> w14
    tunnel: w11 -> [w566]
    tunnel: w10 -> [w565]
    tunnel: [w563] -> w3
    tunnel: [w562] -> w2
    stop <- w583 stop-if-true
    n178 = Tick Count (ms)() -> (millisecond timer value=w580:u32)
    n179 = Dequeue Element(queue=w566, error in (no error)=w565) -> (element=w573:waveform(dbl)[])  [unwired: 1 in, 3 out]
    n180 = control-ref of="stop"() -> (w564:refnum<vi>)
    n181 = Subtract(x=w580, y=w581) -> (x-y=→"Consumer Loop Time / ms":u32)
    n182 = Index Array(array=w573, index=1) -> (element=w570:waveform(dbl))
    n183 = Index Array(array=w573, index=0) -> (element=w569:waveform(dbl))
    n184 = property class="Bool"(reference=w564) -> ("Key Focus"=w583:bool)  [unwired: 1 in, 2 out]
    n185 = call "MS_on_off_sorting.vi"("Laser gate threshold"="Laser gate threshold", "gate_trace"=w570, "Number of sweeps"="Number of Sweeps", "data_trace"=w569, "IR_on_q_error_in"=w576, "IR_on_q_in"=w578, "IR_off_q_error_in"=w577, "IR_off_q_in"=w579) -> ("IR_on_q_error_out"=w574:errorcluster, "IR_on_q_out"=w562:refnum<queue>, "IR_off_q_error_out"=w575:errorcluster, "IR_off_q_out"=w563:refnum<queue>)
  }
  n186 = while {
    tunnel: w45 -> [w598]
    tunnel: w44 -> [w597]
    tunnel: w1 -> [w594]
    tunnel: w43 -> [w593]
    tunnel: [w596] -> w42
    tunnel: [w595] -> w41
    tunnel: [w594] -> w40
    tunnel: [w593] -> w39
    tunnel: w5 -> [w592]
    tunnel: w4 -> [w591]
    tunnel: [w590] -> w36
    tunnel: [w589] -> w35
    stop <- w587 stop-if-true
    n187 = control-ref of="stop"() -> (w586:refnum<vi>)
    n188 = call "get_power_reading.vi"("reference in"=w598, "hDevice"=w594, "channel"=w593, "error in (no error)"=w597) -> ("reference out"=w596:refnum<k7>, "Power / J"=w585:dbl, "error out"=w595:errorcluster)  [unwired: 5 in, 4 out]
    "Power / J" <- w585
    n189 = Greater Than 0?(x=w585) -> (x > 0?=w588:bool)
    n190 = property class="Bool"(reference=w586) -> ("Key Focus"=w587:bool)  [unwired: 1 in, 2 out]
    n191 = case shown="True" w588 {
      tunnel: w592 -> [w600 w605]
      tunnel: w591 -> [w599 w604]
      tunnel: [w600 w603] -> w590
      tunnel: [w599 w602] -> w589
      tunnel: w585 -> [_ w601]
      frame False {
      }
      frame True {
        n192 = Enqueue Element(queue=w605, element=w601, error in (no error)=w604) -> (queue out=w603:refnum<queue>, error out=w602:errorcluster)  [unwired: 1 in, 1 out]
      }
    }
    n193 = Wait (ms)(milliseconds to wait=u32 50) -> ()  [unwired: 1 out]
  }
  n194 = Release Queue(queue=w36, error in (no error)=w35) -> ()  [unwired: 1 in, 3 out]
  n195 = invoke class="ICoLMMeasurement" method="StopStream"(reference=w42, error in=w41, "hDevice"=w40, "channel"=w39) -> (reference out=w47:refnum<k7>, error out=w46:errorcluster)  [unwired: 1 in, 3 out]
  n196 = Release Queue(queue=w3, error in (no error)=w15) -> ()  [unwired: 1 in, 3 out]
  n197 = Release Queue(queue=w2, error in (no error)=w14) -> ()  [unwired: 1 in, 3 out]
  n198 = Close Reference(reference=w47, error in (no error)=w46) -> ()  [unwired: 1 out]
  n199 = call "Close.vi"("error in (no error)"=w24, "VISA resource name"=w25) -> ()  [unwired: 9 in, 1 out]
  n200 = Release Queue(queue=w13, error in (no error)=w12) -> ()  [unwired: 1 in, 3 out]
  n201 = Release Queue(queue=w51, error in (no error)=w50) -> ()  [unwired: 1 in, 3 out]
